vi "Spawn Root.vi"(9 "UID":string, 10 "Actor":refnum<class "Actor.lvclass">) -> (0 "Error out":errorcluster, 5 "Actor out":refnum<class "Actor.lvclass">)   [LabVIEW 2025, in "jettl.lvlib" / "Actor.lvlib"]
uses:
  Actor.lvlib
  Actor/Actor.lvclass
  Core Actor/Core Actor.lvclass
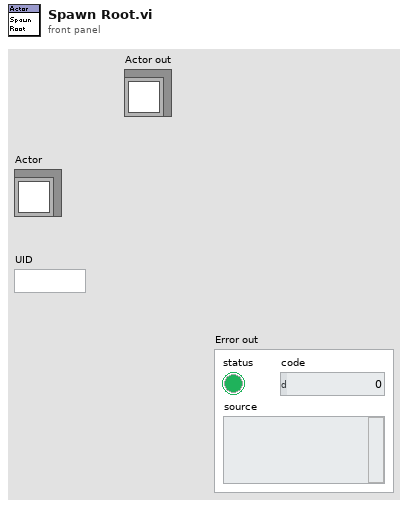
[diagram p1: front panel]
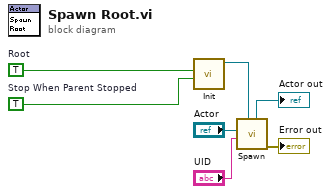
[diagram p0: block diagram]
diagram:
  w1 = TRUE  # Stop When Parent Stopped
  w4 = TRUE  # Root
  n1 = call "Init.vi"("Stop When Parent Stopped"=w1, "Root"=w4) -> ("Core Actor out"=w5:refnum<class "Core Actor.lvclass">)  [unwired: 9 in]
  n2 = call "Spawn.vi"("Actor in"=w5, "UID"="UID", "Actor"="Actor") -> ("Error out"=→"Error out":errorcluster, "Actor out"=→"Actor out":refnum<class "Core Actor.lvclass">)  [unwired: 7 in]
